vi "Configure Power Limits.vi"(0 "VISA resource name":refnum<visa-resource-name>, 5 "Power Low Limit (0 W)":dbl min=0.0 max=4000.0 format="%.1f", 7 "Power High Limit (0 W)":dbl min=0.0 max=4000.0 format="%.1f", 11 "error in (no error)":errorcluster) -> (4 "VISA resource name out":refnum<visa-resource-name>, 15 "error out":errorcluster)   [LabVIEW 2014, in "eec 6700.lvlib"]
doc: "Configures the power limits</B> in the active step of the power source instrument.\n\n<B>Range</B> :0.0~4000 W\n\n0.0 ~500 W - 6705\n0.0 ~1000 W - 6710\n0.0 ~2000 W - 6720\n0.0 ~3000 W - 6730\n0.0 ~4000 W - 6740\n\nPower Limit setting configures a minimum and maximum wattage threshold level. If a minimum wattage level is not reached a failure will occur. If a maximum wattage level is reached the test failure will occur."
uses:
  <instrlib>/eec 6700/eec 6700.lvlib
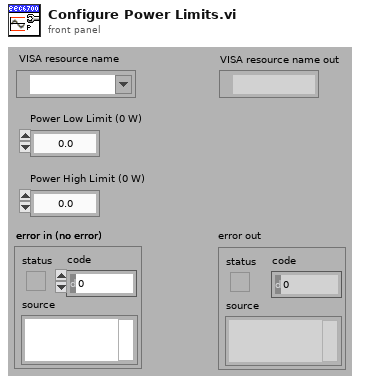
[diagram p1: front panel]
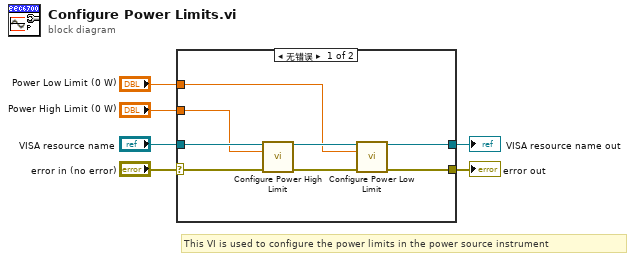
[diagram p0: block diagram]
diagram:
  # "This VI is used to configure the power limits in the power source instrument"
  n1 = case shown="无错误" "error in (no error)" {
    selector: "error in (no error)" -> [w9 w15]
    tunnel: "VISA resource name" -> [w14 w16]
    tunnel: [w12 w15] -> w5
    tunnel: [w11 w16] -> w4
    tunnel: "Power High Limit (0 W)" -> [w8 _]
    tunnel: "Power Low Limit (0 W)" -> [w7 _]
    frame No Error {
      n2 = call <instrlib>:"Configure Power High Limit.vi"("VISA resource name"=w14, "Power High Limit (0 W)"=w8, "error in (no error)"=w9) -> ("VISA resource name out"=w10:refnum<visa-resource-name>, "error out"=w13:errorcluster)  [unwired: 11 in]
      n3 = call <instrlib>:"Configure Power Low Limit.vi"("VISA resource name"=w10, "Power Low Limit (0 W)"=w7, "error in (no error)"=w13) -> ("VISA resource name out"=w11:refnum<visa-resource-name>, "error out"=w12:errorcluster)  [unwired: 11 in]
    }
    frame Error {
    }
  }
  "error out" <- w5
  "VISA resource name out" <- w4
